vi "Read.vi"   [LabVIEW 2009, in "Tektronix DPO MSO 2000 4000 Series.lvlib"]
doc: "Reads waveform data from an oscilloscope. You select to use the <B>Read (Single Waveform)</B> VI if you choose to read waveform from a single channel. You select to use the <B>Read (Multiple Waveforms)</B> VI if you choose to read waveform from on all enabled channels."
uses:
  <instrlib>/Tektronix DPO MSO 2000 4000 Series/Tektronix DPO MSO 2000 4000 Series.lvlib
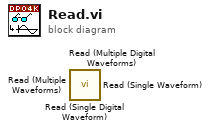
[diagram p0: block diagram]
diagram:
  n1 = call <instrlib>:"Read (Single Digital Waveform).vi"() -> ()  [unwired: 9 in, 3 out]
  n2 = call <instrlib>:"Read (Multiple Digital Waveforms).vi"() -> ()  [unwired: 9 in, 3 out]
  n3 = call <instrlib>:"Read (Multiple Waveforms).vi"() -> ()  [unwired: 9 in, 3 out]
  n4 = call <instrlib>:"Read (Single Waveform).vi"() -> ()  [unwired: 9 in, 3 out]
